vi "Base path.vi"(8 "error in (no error)":errorcluster, 10 "pathList":string[](array[string]), 11 "basePath in":string) -> (0 "error out":errorcluster, 3 "pathArray out":string[](array[string]))   [LabVIEW 2015]
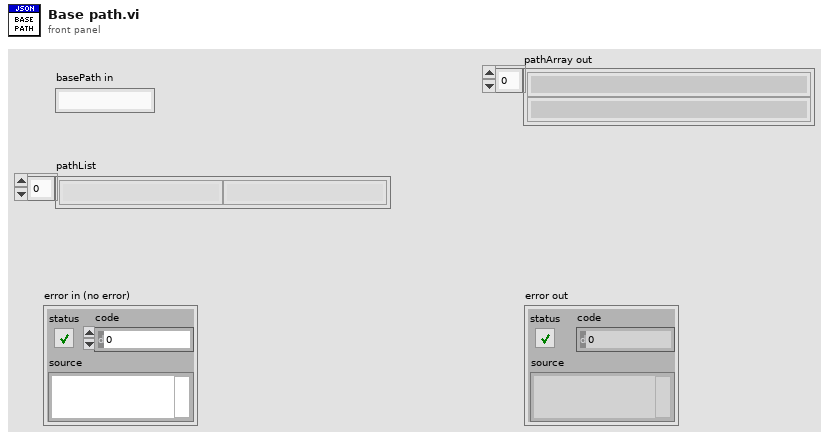
[diagram p1: front panel]
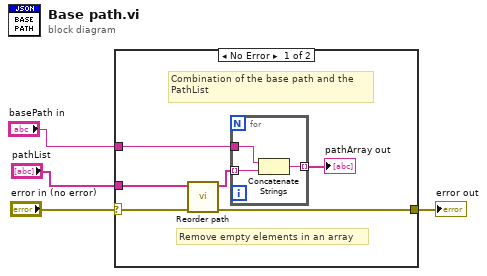
[diagram p0: block diagram]
diagram:
  n1 = case shown="No Error" "error in (no error)" {
    selector: "error in (no error)" -> [w9 w14]
    tunnel: [w8 w14] -> w3
    tunnel: "pathList" -> [w6 _]
    tunnel: "basePath in" -> [w5 _]
    frame No Error {
      # "Remove empty elements in an array"
      # "Combination of the base path and the\nPathList"
      n2 = call "Reorder path.vi"("error in (no error)"=w9, "Array in"=w6) -> ("error out"=w8:errorcluster, "Array out"=w7:string[])  [unwired: 8 in]
      n3 = for {
        tunnel: w7 -> [w12] mode=indexing
        tunnel: w5 -> [w13]
        tunnel: [w11] -> w10 mode=indexing
        n4 = Concatenate Strings(w13, w12) -> (w11:string)
      }
      "pathArray out" <- w10
    }
    frame Error {
    }
  }
  "error out" <- w3
